vi "_RT_CtrlLoop_Pub_Allocator_RS232.vi"(8 "error in (no error)":errorcluster, 11 "RS232ComPort":refnum<class "RS232ComPort.lvclass">) -> (0 "error out":errorcluster)   [LabVIEW 2018]
uses:
  RS232/RS232ComPort.lvclass
  ControlLoop/Laser/Ctl/_ctl_LaserCmd.ctl
  Ctl/_ctl_RT_D999_Settings.ctl
  Ctl/_ctl_RT_SysLog.ctl
  <vilib>/Instr/_visa.llb/VISA Configure Serial Port (Instr).vi
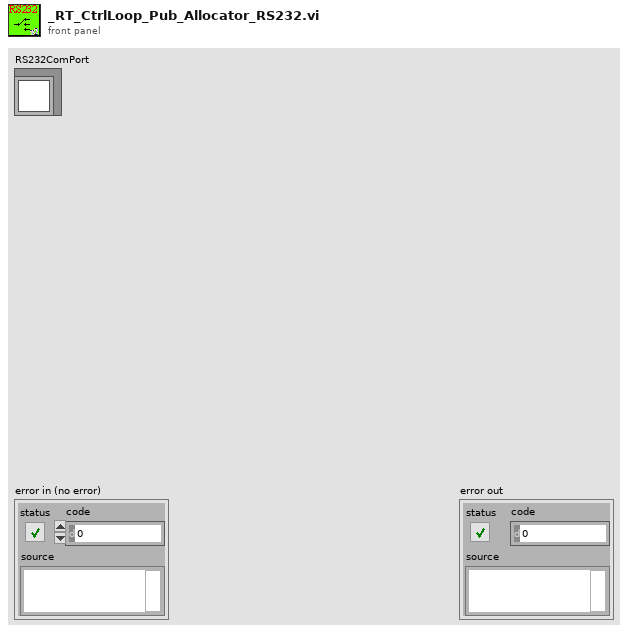
[diagram p1: front panel]
types:
  T1 = typedef "_ctl_RT_SysLog.ctl" = enum16{"None", "Initialize", "StartupRT", "StartupFPGA", "StartupAllocator", "GetMass", "SetWfmCode", "SetLaserCtrl", "SetTurboCtrl", "SetD999Ctrl", "Reconnecting...", "Interrupt", "StopRT"}
  T2 = typedef "_ctl_RT_D999_Settings.ctl" = cluster{"Cmd":enum16{"None", "Init", "Write", "WriteAll", "Read", "ReadAll", "SetEnable", "SetParam", "ReadAO", "ReadSwitch", "ReportID"}, "Variant":variant}
  T3 = typedef "Semaphore RefNum" = refnum<k1>
  T4 = cluster{"Response Str":string, "VISA resource":refnum<visa-resource-name>, "DeviceExist?":bool, "semaphore":T3}
  T5 = typedef "_ctl_LaserCmd.ctl" = enum8{"Diode_On", "Diode_Off", "Standby_On", "Standby_Off", "Internal_Trig", "External_Trig", "Set_Energy", "Set_Frequency", "Read_Version", "Read_STB", "Read_Diode_TEMP", "Read_SHG_TEMP", "Read_THG_TEMP", "Read_Base_Plate_TEMP", "Read_Diode_Hour", "Read_Diode_Maxc", "Read_Diode_Curr", "Read_QSW_CNTS", "Read_PENER", "Read_Freq", "Read_PCUR", "Read_Fault_Codes"}
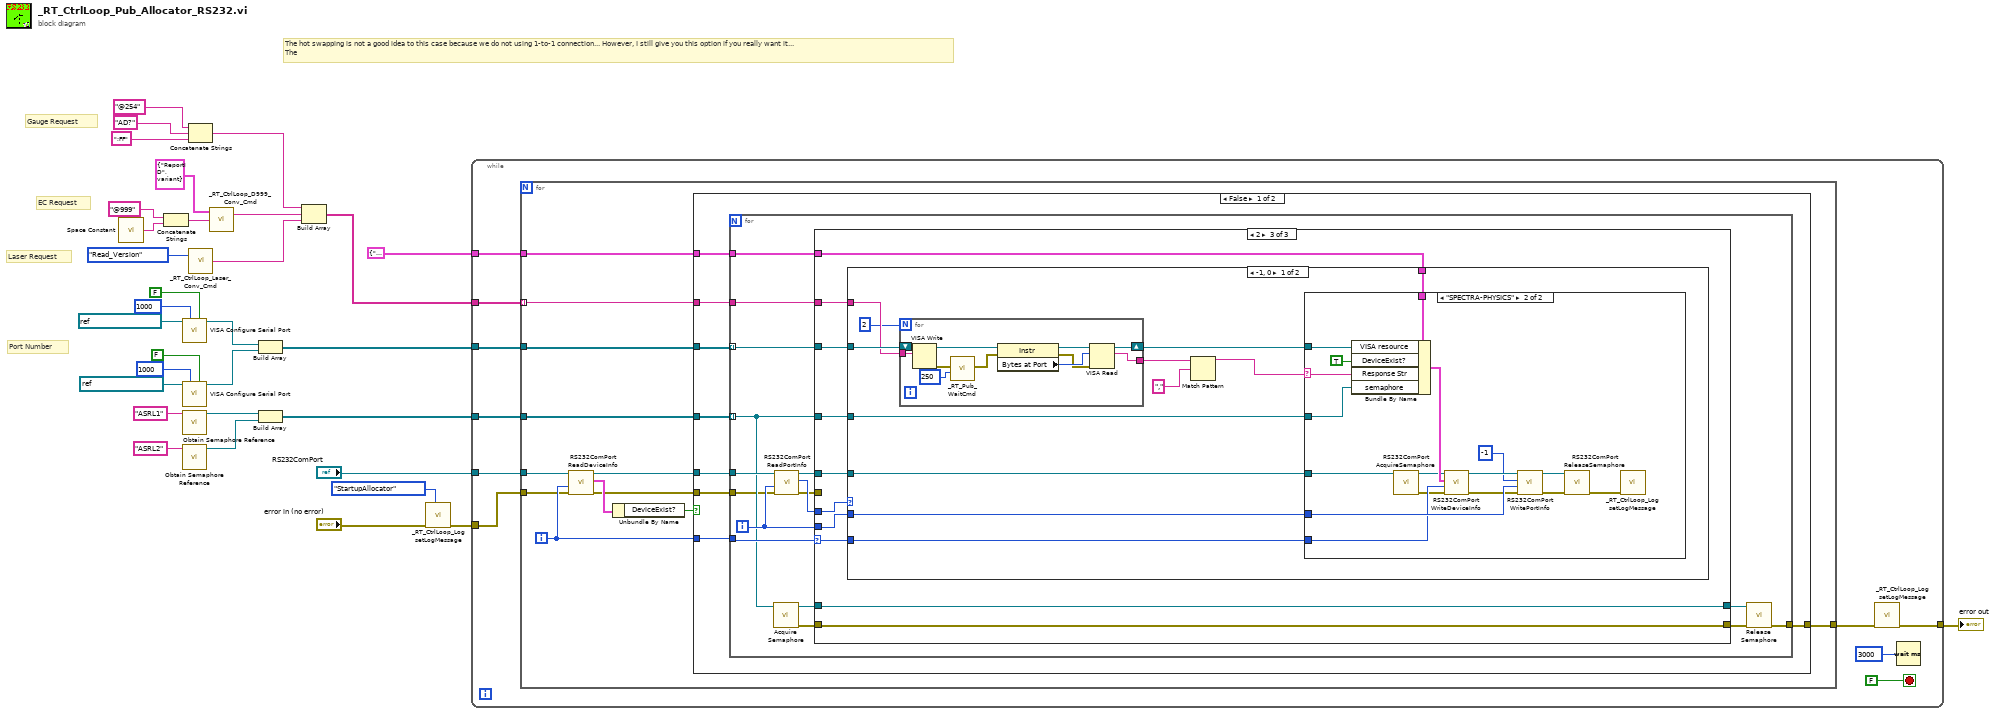
[diagram p0: block diagram]
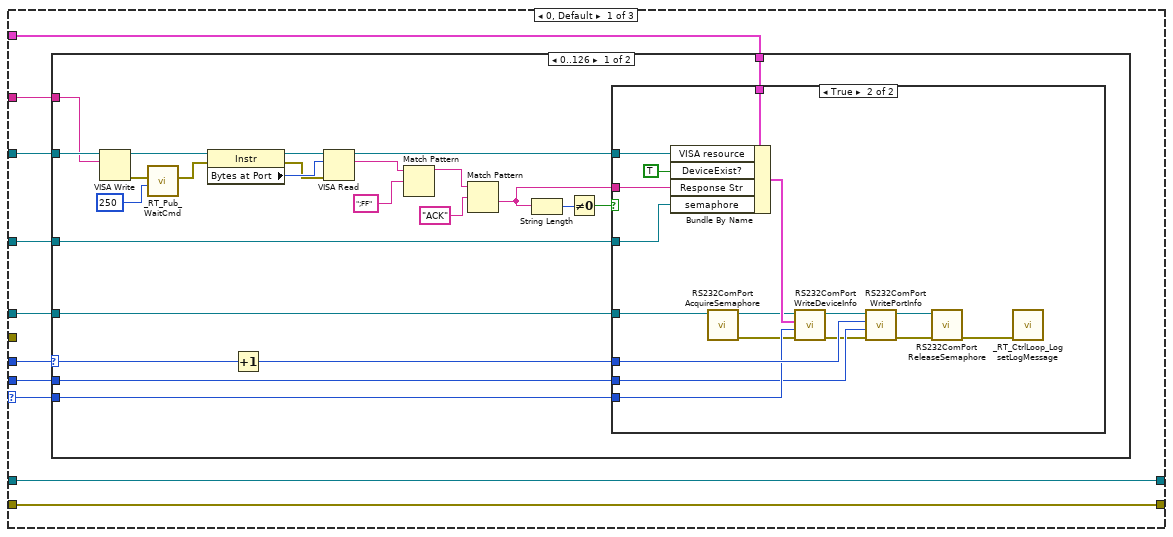
[diagram p2: hidden frame]
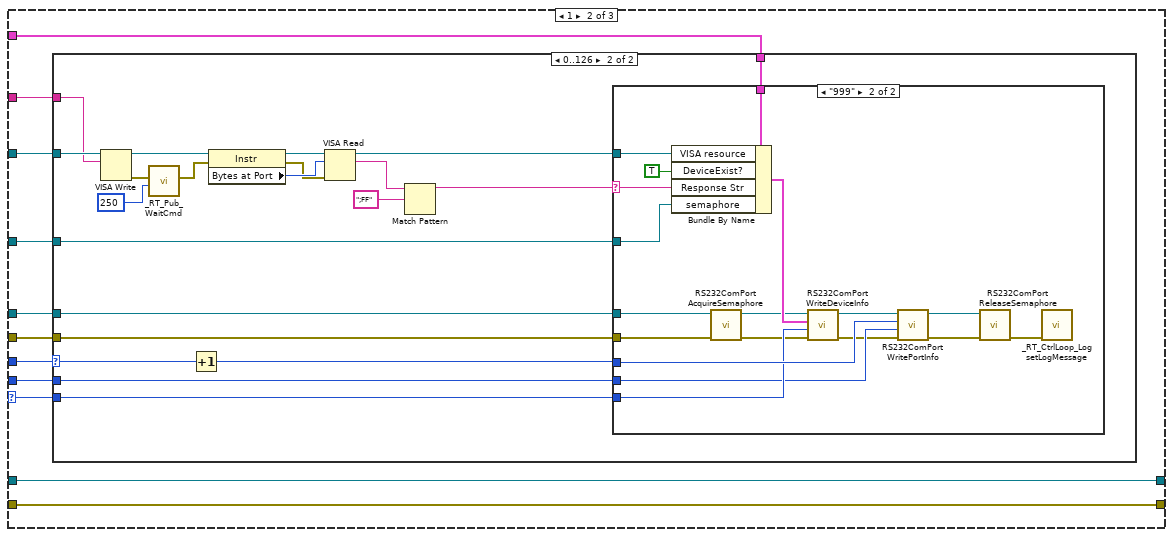
[diagram p5: hidden frame]
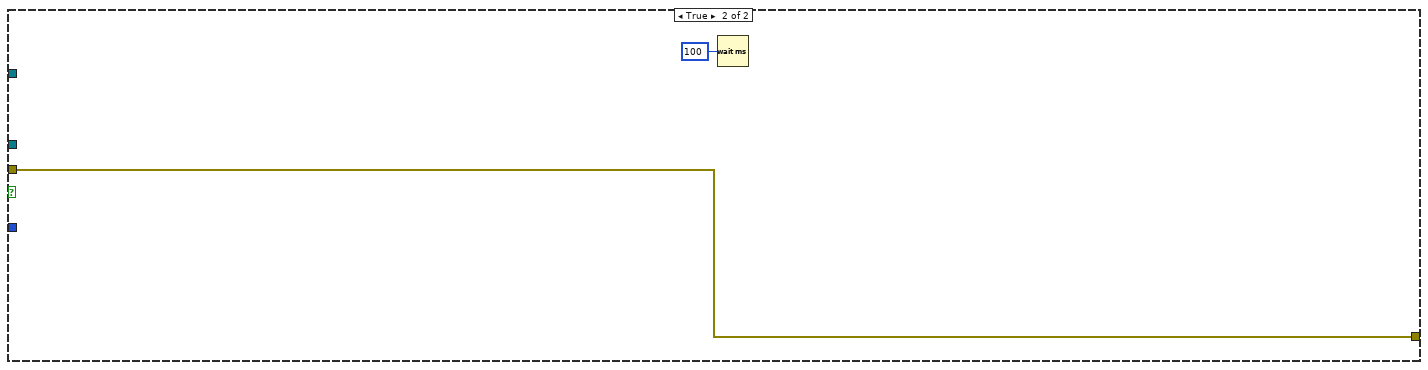
[diagram p10: hidden frame]
diagram:
  # "The hot swapping is not a good idea to this case because we do not using 1-to-1 connection... However, I still give you this option if you really want it...\nThe"
  # "Port Number"
  # "Laser Request"
  # "EC Request"
  # "Gauge Request"
  n1 = call <vilib>:"Space Constant.vi"() -> ("String"=w7:string)
  n2 = Concatenate Strings("@999" ("attention character + addr"), w7) -> (w6:string)
  n3 = call-poly "VISA Configure Serial Port"("VISA resource name"=refnum<visa-resource-name> "ASRL1::INSTR", "timeout (10sec)"=u32 1000, "Enable Termination\nChar (T)"=FALSE ("Enable Termination\nChar (T)")) -> ("VISA resource name out"=w21:refnum<visa-resource-name>)  [unwired: 11 in, 1 out]
  n4 = call-poly "VISA Configure Serial Port"("VISA resource name"=refnum<visa-resource-name> "ASRL2::INSTR", "timeout (10sec)"=u32 1000, "Enable Termination\nChar (T)"=FALSE ("Enable Termination\nChar (T)")) -> ("VISA resource name out"=w20:refnum<visa-resource-name>)  [unwired: 11 in, 1 out]
  n5 = call <vilib>:"Obtain Semaphore Reference.vi"("name (unnamed)"="ASRL1") -> ("semaphore"=w13:T3)  [unwired: 4 in, 2 out]
  n6 = call <vilib>:"Obtain Semaphore Reference.vi"("name (unnamed)"="ASRL2") -> ("semaphore"=w14:T3)  [unwired: 4 in, 2 out]
  n7 = Concatenate Strings("@254" ("attention character + addr"), "AD?" ("string"), ";FF" ("termination")) -> (w18:string)
  n8 = call "_RT_CtrlLoop_Laser_Conv_Cmd.vi"("Command Status"=_ctl_LaserCmd."Read_Version") -> ("Laser Command"=w11:string)  [unwired: 1 in]
  n9 = call "_RT_CtrlLoop_D999_Conv_Cmd.vi"("Head+Addr+Seg"=w6, "CmdParam"=T2 {"Cmd"=enum."ReportID", "Variant"=variant}) -> ("Cmd_String"=w5:string)  [unwired: 1 in, 1 out]
  n10 = Build Array(w21, w20) -> (w19:refnum<visa-resource-name>[])
  n11 = Build Array(w13, w14) -> (w12:T3[])
  n12 = Build Array(w18, w5, w11) -> (w28:string[])
  n13 = call "_RT_CtrlLoop_Log setLogMessage.vi"("system type"=_ctl_RT_SysLog."StartupAllocator", "error in"="error in (no error)") -> ("error out"=w3:errorcluster)  [unwired: 8 in, 1 out]
  n14 = while {
    tunnel: w28 -> [w42]
    tunnel: w19 -> [w41]
    tunnel: T4 {"Response Str"="", "VISA resource"="", "DeviceExist?"=FALSE, "semaphore"=refnum} ("Type") -> [w40]
    tunnel: w12 -> [w39]
    tunnel: "RS232ComPort" -> [w37]
    tunnel: w3 -> [w35]
    tunnel: [w33] -> w2
    stop <- FALSE stop-if-true
    n15 = for {
      tunnel: w42 -> [w54] mode=indexing
      tunnel: w41 -> [w53]
      tunnel: w40 -> [w52]
      tunnel: w39 -> [w51]
      tunnel: w37 -> [w49]
      tunnel: w35 -> [w44]
      tunnel: [w43] -> w34
      i -> [w48]
      n16 = call-dynamic "RS232ComPort ReadDeviceInfo.vi"("error in (no error)"=w44, "DeviceIndex"=w48, "RS232ComPort in"=w49) -> ("error out"=w45:errorcluster, "DeviceInfo"=w47:T4, "RS232ComPort out"=w46:refnum<class "RS232ComPort.lvclass">)  [unwired: 6 in]
      n17 = Unbundle By Name(w47) -> ("DeviceExist?"=w50:bool)
      n18 = case shown="False" w50 {
        tunnel: w54 -> [w62 _]
        tunnel: w53 -> [w61 _]
        tunnel: w52 -> [w60 _]
        tunnel: w51 -> [w59 _]
        tunnel: w48 -> [w58 _]
        tunnel: w46 -> [w57 _]
        tunnel: w45 -> [w56 w230]
        tunnel: [w55 w230] -> w43
        frame False {
          n19 = for {
            tunnel: w62 -> [w75]
            tunnel: w61 -> [w77] mode=indexing
            tunnel: w58 -> [w78]
            tunnel: w60 -> [w76]
            tunnel: w59 -> [w70] mode=indexing
            tunnel: w57 -> [w74]
            tunnel: w56 -> [w65]
            tunnel: [w63] -> w55
            i -> [w71]
            n20 = call <vilib>:"Acquire Semaphore.vi"("semaphore"=w70) -> ("error out"=w69:errorcluster, "semaphore out"=w66:T3)  [unwired: 4 in, 1 out]
            n21 = call-dynamic "RS232ComPort ReadPortInfo.vi"("error in (no error)"=w65, "Channel"=w71, "RS232ComPort in"=w74) -> ("error out"=w64:errorcluster, "Status"=w73:i8, "RS232ComPort out"=w72:refnum<class "RS232ComPort.lvclass">)  [unwired: 6 in]
            n22 = case shown="2" w78 {
              selector: w78 -> [w87 w139 w188]
              tunnel: w70 -> [w85 w137 w186]
              tunnel: w77 -> [w88 w140 w189]
              tunnel: w76 -> [w86 w138 w187]
              tunnel: w75 -> [w82 w134 w183]
              tunnel: w73 -> [w84 w136 w185]
              tunnel: w72 -> [w83 w135 w184]
              tunnel: w71 -> [w81 w133 w182]
              tunnel: w69 -> [w80 w131 w181]
              tunnel: [w80 w131 w181] -> w68
              tunnel: [w79 w132 w180] -> w67
              tunnel: w66 -> [w79 w132 w180]
              tunnel: w64 -> [_ w130 _]
              frame 0, Default {
                n23 = case shown="0..126" w84 {
                  selector: w84 -> [w91 _]
                  tunnel: w88 -> [w105 _]
                  tunnel: w87 -> [w98 _]
                  tunnel: w86 -> [w95 _]
                  tunnel: w85 -> [w94 _]
                  tunnel: w83 -> [w93 _]
                  tunnel: w82 -> [w92 _]
                  tunnel: w81 -> [w89 _]
                  frame 0..126 {
                    n24 = VISA Write(VISA resource name=w105, write buffer=w92) -> (VISA resource name out=w109:refnum<visa-resource-name>, error out=w106:errorcluster)  [unwired: 1 in, 1 out]
                    n25 = call "_RT_Pub_WaitCmd.vi"("milliseconds to wait"=u32 250, "error in (no error)"=w106) -> ("error out"=w108:errorcluster)  [unwired: 9 in]
                    n26 = property class="Instr"(reference=w109, error in=w108) -> (reference out=w112:refnum<visa-resource-name>, error out=w110:errorcluster, "Bytes at Port"=w111:u32)
                    n27 = Increment(x=w91) -> (x+1=w90:i8)
                    n28 = VISA Read(VISA resource name=w112, byte count=w111, error in (no error)=w110) -> (VISA resource name out=w96:refnum<visa-resource-name>, read buffer=w99:string)  [unwired: 2 out]
                    n29 = Match Pattern(string=w99, regular expression=";FF") -> (before substring=w97:string)  [unwired: 1 in, 3 out]
                    n30 = Match Pattern(string=w97, regular expression="ACK") -> (after substring=w104:string)  [unwired: 1 in, 3 out]
                    n31 = String Length(string=w104) -> (length=w101:i32)
                    n32 = Not Equal To 0?(x=w101) -> (x != 0?=w103:bool)
                    n33 = case shown="True" w103 {
                      tunnel: w104 -> [_ w128]
                      tunnel: w98 -> [_ w121]
                      tunnel: w96 -> [_ w127]
                      tunnel: w95 -> [_ w126]
                      tunnel: w94 -> [_ w125]
                      tunnel: w93 -> [_ w119]
                      tunnel: w90 -> [_ w122]
                      tunnel: w89 -> [_ w120]
                      frame False {
                      }
                      frame True {
                        n34 = Bundle By Name(cluster=w126, "VISA resource"=w127, "DeviceExist?"=TRUE, "Response Str"=w128, "semaphore"=w125) -> (w124:T4)
                        n35 = call-dynamic "RS232ComPort AcquireSemaphore.vi"("RS232ComPort in"=w119) -> ("error out"=w114:errorcluster, "RS232ComPort out"=w118:refnum<class "RS232ComPort.lvclass">)  [unwired: 9 in]
                        n36 = call-dynamic "RS232ComPort WriteDeviceInfo.vi"("error in (no error)"=w114, "DeviceIndex"=w121, "DeviceInfo"=w124, "RS232ComPort in"=w118) -> ("error out"=w115:errorcluster, "RS232ComPort out"=w123:refnum<class "RS232ComPort.lvclass">)  [unwired: 6 in]
                        n37 = call-dynamic "RS232ComPort WritePortInfo.vi"("error in (no error)"=w115, "Channel"=w120, "Status"=w122, "RS232ComPort in"=w123) -> ("error out"=w116:errorcluster, "RS232ComPort out"=w117:refnum<class "RS232ComPort.lvclass">)  [unwired: 6 in]
                        n38 = call-dynamic "RS232ComPort ReleaseSemaphore.vi"("error in (no error)"=w116, "RS232ComPort in"=w117) -> ("error out"=w113:errorcluster)  [unwired: 8 in, 1 out]
                        n39 = call "_RT_CtrlLoop_Log setLogMessage.vi"("error in"=w113) -> ()  [unwired: 9 in, 2 out]
                      }
                    }
                  }
                  frame Default {
                  }
                }
              }
              frame 1 {
                n40 = case shown="0..126" w136 {
                  selector: w136 -> [_ w144]
                  tunnel: w140 -> [_ w154]
                  tunnel: w139 -> [_ w151]
                  tunnel: w138 -> [_ w149]
                  tunnel: w137 -> [_ w148]
                  tunnel: w135 -> [_ w147]
                  tunnel: w134 -> [_ w146]
                  tunnel: w133 -> [_ w142]
                  tunnel: w130 -> [_ w141]
                  frame Default {
                  }
                  frame 0..126 {
                    n41 = VISA Write(VISA resource name=w154, write buffer=w146) -> (VISA resource name out=w158:refnum<visa-resource-name>, error out=w155:errorcluster)  [unwired: 1 in, 1 out]
                    n42 = call "_RT_Pub_WaitCmd.vi"("milliseconds to wait"=u32 250, "error in (no error)"=w155) -> ("error out"=w157:errorcluster)  [unwired: 9 in]
                    n43 = Increment(x=w144) -> (x+1=w143:i8)
                    n44 = property class="Instr"(reference=w158, error in=w157) -> (reference out=w161:refnum<visa-resource-name>, error out=w159:errorcluster, "Bytes at Port"=w160:u32)
                    n45 = VISA Read(VISA resource name=w161, byte count=w160, error in (no error)=w159) -> (VISA resource name out=w150:refnum<visa-resource-name>, read buffer=w152:string)  [unwired: 2 out]
                    n46 = Match Pattern(string=w152, regular expression=";FF") -> (before substring=w145:string)  [unwired: 1 in, 3 out]
                    n47 = case shown="\"999\"" w145 {
                      selector: w145 -> [_ w173]
                      tunnel: w151 -> [_ w171]
                      tunnel: w150 -> [_ w178]
                      tunnel: w149 -> [_ w177]
                      tunnel: w148 -> [_ w176]
                      tunnel: w147 -> [_ w168]
                      tunnel: w143 -> [_ w172]
                      tunnel: w142 -> [_ w170]
                      tunnel: w141 -> [_ w163]
                      frame "False", Default {
                      }
                      frame "999" {
                        n48 = Bundle By Name(cluster=w177, "VISA resource"=w178, "DeviceExist?"=TRUE, "Response Str"=w173, "semaphore"=w176) -> (w175:T4)
                        n49 = call-dynamic "RS232ComPort AcquireSemaphore.vi"("error in (no error)"=w163, "RS232ComPort in"=w168) -> ("error out"=w166:errorcluster, "RS232ComPort out"=w167:refnum<class "RS232ComPort.lvclass">)  [unwired: 8 in]
                        n50 = call-dynamic "RS232ComPort WriteDeviceInfo.vi"("error in (no error)"=w166, "DeviceIndex"=w171, "DeviceInfo"=w175, "RS232ComPort in"=w167) -> ("error out"=w165:errorcluster, "RS232ComPort out"=w174:refnum<class "RS232ComPort.lvclass">)  [unwired: 6 in]
                        n51 = call-dynamic "RS232ComPort WritePortInfo.vi"("error in (no error)"=w165, "Channel"=w170, "Status"=w172, "RS232ComPort in"=w174) -> ("error out"=w164:errorcluster, "RS232ComPort out"=w169:refnum<class "RS232ComPort.lvclass">)  [unwired: 6 in]
                        n52 = call-dynamic "RS232ComPort ReleaseSemaphore.vi"("error in (no error)"=w164, "RS232ComPort in"=w169) -> ("error out"=w162:errorcluster)  [unwired: 8 in, 1 out]
                        n53 = call "_RT_CtrlLoop_Log setLogMessage.vi"("error in"=w162) -> ()  [unwired: 9 in, 2 out]
                      }
                    }
                  }
                }
              }
              frame 2 {
                n54 = case shown="-1, 0" w185 {
                  tunnel: w189 -> [w201 _]
                  tunnel: w188 -> [w199 _]
                  tunnel: w187 -> [w197 _]
                  tunnel: w186 -> [w196 _]
                  tunnel: w184 -> [w195 _]
                  tunnel: w183 -> [w194 _]
                  tunnel: w182 -> [w190 _]
                  frame -1, 0 {
                    n55 = for {
                      N: 2 -> [_]
                      tunnel: [w204] -> w200
                      tunnel: w194 -> [w202]
                      shift-right: [w203] -> w198
                      shift-left: w201 -> [w205]
                      n56 = VISA Write(VISA resource name=w205, write buffer=w202) -> (VISA resource name out=w209:refnum<visa-resource-name>, error out=w206:errorcluster)  [unwired: 1 in, 1 out]
                      n57 = call "_RT_Pub_WaitCmd.vi"("milliseconds to wait"=u32 250, "error in (no error)"=w206) -> ("error out"=w208:errorcluster)  [unwired: 9 in]
                      n58 = property class="Instr"(reference=w209, error in=w208) -> (reference out=w212:refnum<visa-resource-name>, error out=w210:errorcluster, "Bytes at Port"=w211:u32)
                      n59 = VISA Read(VISA resource name=w212, byte count=w211, error in (no error)=w210) -> (VISA resource name out=w203:refnum<visa-resource-name>, read buffer=w204:string)  [unwired: 2 out]
                    }
                    n60 = Match Pattern(string=w200, regular expression=",") -> (before substring=w193:string)  [unwired: 1 in, 3 out]
                    n61 = case shown="\"SPECTRA-PHYSICS\"" w193 {
                      selector: w193 -> [_ w222]
                      tunnel: w199 -> [_ w223]
                      tunnel: w198 -> [_ w228]
                      tunnel: w197 -> [_ w227]
                      tunnel: w196 -> [_ w214]
                      tunnel: w195 -> [_ w220]
                      tunnel: w190 -> [_ w224]
                      frame "False", Default {
                      }
                      frame "SPECTRA-PHYSICS" {
                        n62 = Bundle By Name(cluster=w227, "VISA resource"=w228, "DeviceExist?"=TRUE, "Response Str"=w222, "semaphore"=w214) -> (w226:T4)
                        n63 = call-dynamic "RS232ComPort AcquireSemaphore.vi"("RS232ComPort in"=w220) -> ("error out"=w218:errorcluster, "RS232ComPort out"=w219:refnum<class "RS232ComPort.lvclass">)  [unwired: 9 in]
                        n64 = call-dynamic "RS232ComPort WriteDeviceInfo.vi"("error in (no error)"=w218, "DeviceIndex"=w223, "DeviceInfo"=w226, "RS232ComPort in"=w219) -> ("error out"=w215:errorcluster, "RS232ComPort out"=w225:refnum<class "RS232ComPort.lvclass">)  [unwired: 6 in]
                        n65 = call-dynamic "RS232ComPort WritePortInfo.vi"("error in (no error)"=w215, "Channel"=w224, "Status"=i8 -1, "RS232ComPort in"=w225) -> ("error out"=w216:errorcluster, "RS232ComPort out"=w217:refnum<class "RS232ComPort.lvclass">)  [unwired: 6 in]
                        n66 = call-dynamic "RS232ComPort ReleaseSemaphore.vi"("error in (no error)"=w216, "RS232ComPort in"=w217) -> ("error out"=w213:errorcluster)  [unwired: 8 in, 1 out]
                        n67 = call "_RT_CtrlLoop_Log setLogMessage.vi"("error in"=w213) -> ()  [unwired: 9 in, 2 out]
                      }
                    }
                  }
                  frame Default {
                  }
                }
              }
            }
            n68 = call <vilib>:"Release Semaphore.vi"("error in (no error)"=w68, "semaphore"=w67) -> ("error out"=w63:errorcluster)  [unwired: 4 in, 1 out]
          }
        }
        frame True {
          n69 = Wait (ms)(milliseconds to wait=u32 100) -> ()  [unwired: 1 out]
        }
      }
    }
    n70 = call "_RT_CtrlLoop_Log setLogMessage.vi"("error in"=w34) -> ("error out"=w33:errorcluster)  [unwired: 9 in, 1 out]
    n71 = Wait (ms)(milliseconds to wait=u32 3000) -> ()  [unwired: 1 out]
  }
  "error out" <- w2
